vi "_CSTK_Button_Icon_CreateBGImage.vi"(0 "按钮大小":T6={"Width"=100, "Height"=30} caption="控件大小", 1 "LOGO图片数据":T5, 2 "LOGO属性":T4, 5 "背景颜色":u32(colorbox)=9567230, 7 "边框颜色":u32(colorbox)=12237498, 9 "边框属性":T1={"Radius"=0, "Border Style"={"Width"=3, "Style"=enum."Solid"}}, 12 "布尔文本":string, 13 "文本属性":T2) -> (4 "图像输出":picture, 6 "绘图区域大小":T6={"Width"=101, "Height"=31}, 8 "字符串起始坐标":i16)   [LabVIEW 2015, in "CSTK_Button_Icon.xctl"]
uses:
  CSTK_Button_Icon.xctl
  <vilib>/Utility/miscctls.llb/LVBoundsTypeDef.ctl
  <vilib>/picture/picture.llb/imagedata.ctl
  TypeDefinitions/_CSTK_Button_Icon_LogoProperties_Data.ctl
  TypeDefinitions/_CSTK_Button_Icon_TextProperties_Data.ctl
  TypeDefinitions/_CSTK_Button_Icon_TextProperties_FontStyle.ctl
  TypeDefinitions/_CSTK_Button_Icon_BorderProperties_Data.ctl
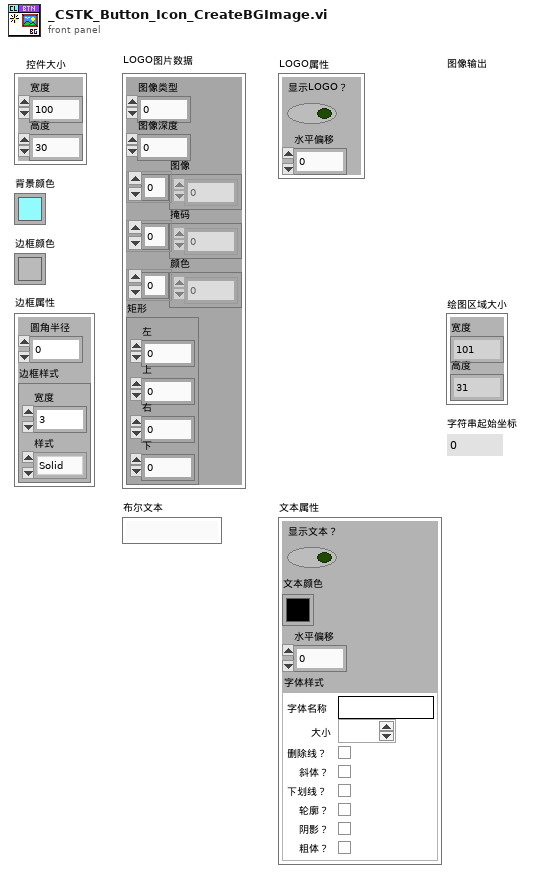
[diagram p1: front panel]
types:
  T1 = typedef "CSTK_Button_Icon.xctl/_CSTK_Button_Icon_BorderProperties_Data.ctl" = cluster{"Radius":i16, "Border Style":cluster{"Width":u16, "Style":enum32{"Solid", "Dash", "Dot", "DashDot", "DashDotDot"}}}
  T2 = typedef "CSTK_Button_Icon.xctl/_CSTK_Button_Icon_TextProperties_Data.ctl" = cluster{"Display Text?":bool, "Text Color":u32, "Horizontal Offset":i16, "Font Style":T3}
  T3 = typedef "CSTK_Button_Icon.xctl/_CSTK_Button_Icon_TextProperties_FontStyle.ctl" = cluster{"Font Name":string, "Size":i16, "Strikeout?":bool, "Italic?":bool, "Underline?":bool, "Outline?":bool, "Shadow?":bool, "Bold?":bool}
  T4 = typedef "CSTK_Button_Icon.xctl/_CSTK_Button_Icon_LogoProperties_Data.ctl" = cluster{"Display Logo?":bool, "Horizontal Offset":i16}
  T5 = typedef "imagedata.ctl" = cluster{"image type":i32, "image depth":i32, "image":u8[], "mask":u8[], "colors":u32[], "Rectangle":cluster{"left":i16, "top":i16, "right":i16, "bottom":i16}}
  T6 = typedef "LVBoundsTypeDef.ctl" = cluster{"Width":u32, "Height":u32}
  T7 = cluster{"left":i16, "top":i16, "right":i16, "bottom":i16}
  T8 = cluster{"Width":u16, "Style":enum32{"Solid", "Dash", "Dot", "DashDot", "DashDotDot"}}
  T9 = enum16{"User-specified Font", "Application Font", "System Font", "Dialog Font"}
  T10 = cluster{"horizontal":enum16{"left", "center", "right"}, "vertical":enum16{"top", "center", "bottom"}}
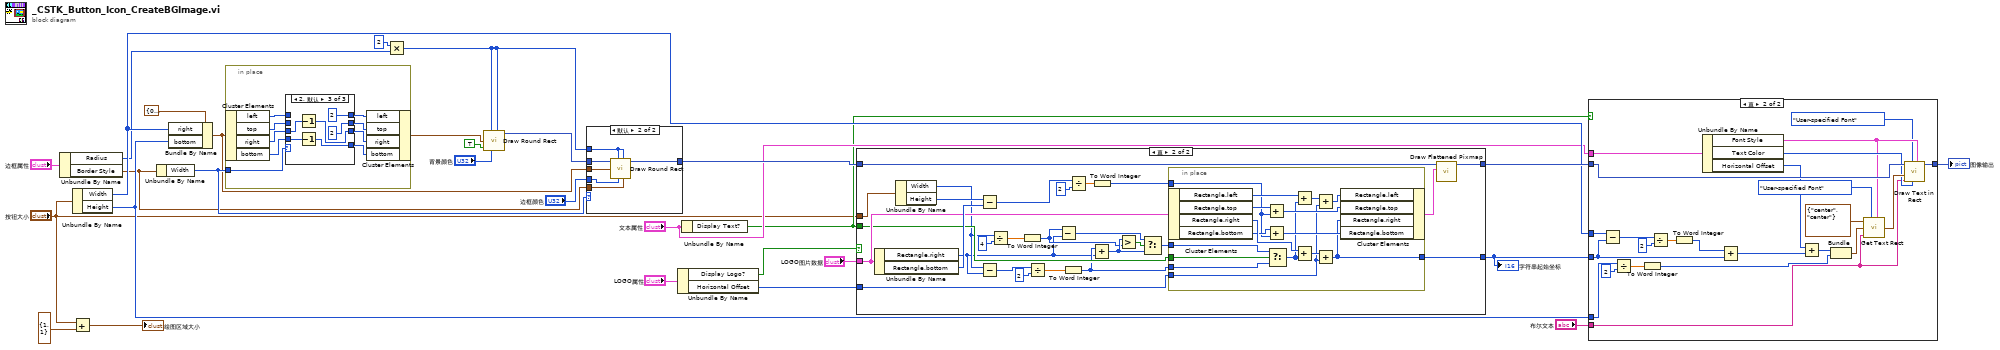
[diagram p0: block diagram]
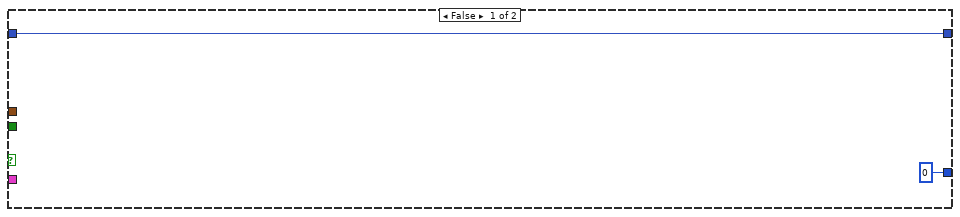
[diagram p3: hidden frame]
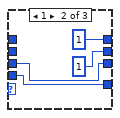
[diagram p6: hidden frame]
diagram:
  n1 = Unbundle By Name("边框属性") -> ("Radius"=w4:i16, "Border Style"=w3:T8)
  n2 = Unbundle By Name("按钮大小") -> ("Width"=w10:u32, "Height"=w9:u32)
  n3 = Add(x="按钮大小", y=T6 {"Width"=1, "Height"=1}) -> (x+y=→"绘图区域大小":T6)
  n4 = Unbundle By Name(w3) -> ("Width"=w21:u16)
  n5 = Bundle By Name(cluster=T7 {"left"=0, "top"=0, "right"=0, "bottom"=0} ("rect"), "right"=w10, "bottom"=w9) -> (w20:T7)
  n6 = in-place {
    in-place-border: w21 -> [w32]
    n7 = in-place-cluster #1(w20) -> ("left"=w31:i16, "top"=w30:i16, "right"=w36:i16, "bottom"=w34:i16)
    n8 = case shown="2, 默认" w32 {
      tunnel: [w42 i16 1 ("left") i16 2 ("left")] -> w38
      tunnel: [w41 i16 1 ("top") i16 2 ("top")] -> w37
      tunnel: w36 -> [w40 w44 w50]
      tunnel: [w40 w44 w49] -> w35
      tunnel: w34 -> [w39 w43 w48]
      tunnel: [w39 w43 w47] -> w33
      tunnel: w31 -> [w42 _ _]
      tunnel: w30 -> [w41 _ _]
      frame 0 {
      }
      frame 1 {
      }
      frame 2, Default {
        n9 = Decrement(x=w50) -> (x-1=w49:i16)
        n10 = Decrement(x=w48) -> (x-1=w47:i16)
      }
    }
    n11 = in-place-cluster #1("left"=w38, "top"=w37, "right"=w35, "bottom"=w33) -> (w25:T7)
  }
  n12 = Multiply(x=i16 2, y=w4) -> (x*y=w23:i16)
  n13 = call <vilib>:"Draw Round Rect.vi"("oval width"=w23, "rect"=w25, "fill?(F)"=TRUE, "color(black)"="背景颜色", "oval height"=w23) -> ("new picture"=w27:picture)  [unwired: 4 in]
  n14 = case shown="默认" w21 {
    tunnel: "边框颜色" -> [_ w59]
    tunnel: w27 -> [w53 w58]
    tunnel: w23 -> [_ w57]
    tunnel: [w53 w56] -> w17
    tunnel: w20 -> [_ w55]
    tunnel: w3 -> [_ w54]
    frame 0 {
    }
    frame Default {
      n15 = call <vilib>:"Draw Round Rect.vi"("picture"=w58, "oval width"=w57, "rect"=w55, "color(black)"=w59, "oval height"=w57, "pen"=w54) -> ("new picture"=w56:picture)  [unwired: 3 in]
    }
  }
  n16 = Unbundle By Name("LOGO属性") -> ("Display Logo?"=w14:bool, "Horizontal Offset"=w13:i16)
  n17 = Unbundle By Name("文本属性") -> ("Display Text?"=w2:bool)
  n18 = case shown="真" w14 {
    tunnel: w17 -> [w61 w88]
    tunnel: [w61 w87] -> w12
    tunnel: "LOGO图片数据" -> [_ w82]
    tunnel: w13 -> [_ w79]
    tunnel: [i16 0 w78] -> w7
    tunnel: w2 -> [_ w72]
    tunnel: "按钮大小" -> [_ w77]
    frame False {
    }
    frame True {
      n19 = Unbundle By Name(w82) -> ("Rectangle.right"=w63:i16, "Rectangle.bottom"=w86:i16)
      n20 = Unbundle By Name(w77) -> ("Width"=w71:u32, "Height"=w76:u32)
      n21 = Subtract(x=w76, y=w86) -> (x-y=w85:u32)
      n22 = Subtract(x=w71, y=w63) -> (x-y=w73:u32)
      n23 = Divide(x=w71, y=u32 4) -> (x/y=w69:dbl)
      n24 = To Word Integer(number=w69) -> (16bit integer=w64:i16)
      n25 = Divide(x=w73, y=u32 2) -> (x/y=w74:dbl)
      n26 = Subtract(x=w64, y=w63) -> (x-y=w62:i16)
      n27 = To Word Integer(number=w74) -> (16bit integer=w68:i16)
      n28 = Divide(x=w85, y=u32 2) -> (x/y=w83:dbl)
      n29 = To Word Integer(number=w83) -> (16bit integer=w81:i16)
      n30 = Add(x=w68, y=w63) -> (x+y=w66:i16)
      n31 = Greater?(x=w66, y=w64) -> (0:w67:bool)
      n32 = Select(t=w62, s=w67, f=w66) -> (s? t:f=w65:i16)
      n33 = in-place {
        in-place-border: w81 -> [w96]
        in-place-border: w79 -> [w94]
        in-place-border: [w93] -> w78
        in-place-border: w68 -> [w90]
        in-place-border: w72 -> [w92]
        in-place-border: w65 -> [w89]
        n34 = in-place-cluster #2(w82) -> ("Rectangle.left"=w104:i16, "Rectangle.top"=w99:i16, "Rectangle.right"=w98:i16, "Rectangle.bottom"=w97:i16)
        n35 = Add(x=w99, y=w96) -> (x+y=w102:i16)
        n36 = Add(x=w97, y=w96) -> (x+y=w100:i16)
        n37 = Select(t=w89, s=w92, f=w90) -> (s? t:f=w91:i16)
        n38 = Add(x=w104, y=w91) -> (x+y=w103:i16)
        n39 = Add(x=w98, y=w91) -> (x+y=w101:i16)
        n40 = Add(x=w103, y=w94) -> (x+y=w95:i16)
        n41 = Add(x=w101, y=w94) -> (x+y=w93:i16)
        n42 = in-place-cluster #2("Rectangle.left"=w95, "Rectangle.top"=w102, "Rectangle.right"=w93, "Rectangle.bottom"=w100) -> (w80:T5)
      }
      n43 = call <vilib>:"Draw Flattened Pixmap.vi"("image data"=w80, "picture"=w88) -> ("new picture"=w87:picture)  [unwired: 7 in]
    }
  }
  "字符串起始坐标" <- w7
  n44 = case shown="真" w2 {
    tunnel: w12 -> [w105 w129]
    tunnel: [w105 w128] -> w11
    tunnel: w10 -> [_ w127]
    tunnel: w7 -> [_ w123]
    tunnel: w9 -> [_ w121]
    tunnel: "布尔文本" -> [_ w110]
    tunnel: "文本属性" -> [_ w114]
    frame False {
    }
    frame True {
      n45 = Subtract(x=w127, y=w123) -> (x-y=w126:u32)
      n46 = Divide(x=w121, y=u32 2) -> (x/y=w119:dbl)
      n47 = To Word Integer(number=w119) -> (16bit integer=w117:i16)
      n48 = Divide(x=w126, y=u32 2) -> (x/y=w124:dbl)
      n49 = To Word Integer(number=w124) -> (16bit integer=w122:i16)
      n50 = Unbundle By Name(w114) -> ("Font Style"=w111:T3, "Text Color"=w112:u32, "Horizontal Offset"=w108:i16)
      n51 = Add(x=w122, y=w123) -> (x+y=w118:i16)
      n52 = Add(x=w108, y=w118) -> (x+y=w109:i16)
      n53 = Bundle(w109, w117) -> (w115:cluster{i16, i16})  [unwired: 1 in]
      n54 = call <vilib>:"Get Text Rect.vi"("alignment(left, top)"=T10 {"horizontal"=enum."center", "vertical"=enum."center"}, "desired font(Application)"=T9."User-specified Font", "origin(0,0)"=w115, "text"=w110, "[user-specified font]"=w111) -> ("rect"=w113:T7)  [unwired: 4 in]
      n55 = call <vilib>:"Draw Text in Rect.vi"("[user-specified font]"=w111, "text color(black)"=w112, "desired font(Application)"=T9."User-specified Font", "text"=w110, "rect"=w113, "picture"=w129) -> ("new picture"=w128:picture)  [unwired: 5 in]
    }
  }
  "图像输出" <- w11
